vi "Shift left right.vi"(0 "TETRIS BLOCK":u8[][](array[numeric]), 1 "Filled Array":u8[][](array[numeric]), 2 "Move Right":bool) -> (7 "After Shift":u8[][](array[numeric]))   [LabVIEW 2018]
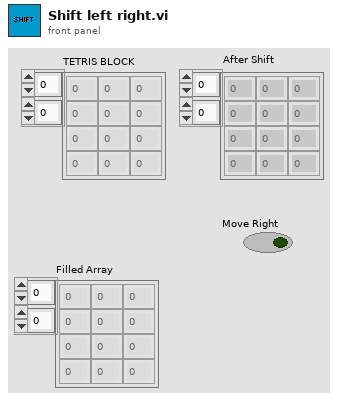
[diagram p1: front panel]
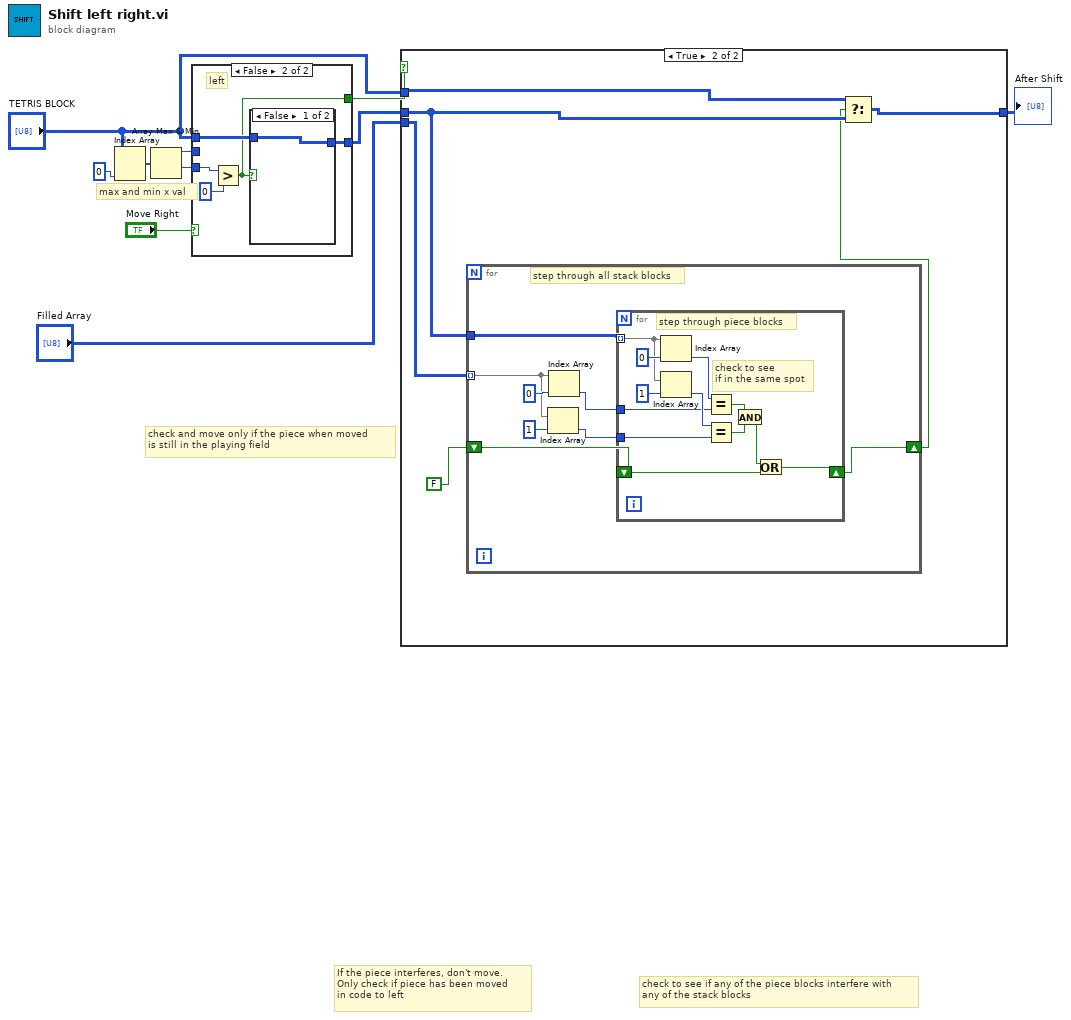
[diagram p0: block diagram]
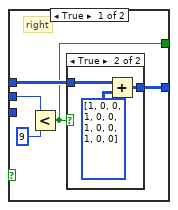
[diagram p3: hidden frame]
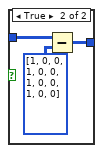
[diagram p5: hidden frame]
diagram:
  # "check to see if any of the piece blocks interfere with \nany of the stack blocks"
  # "max and min x val"
  # "If the piece interferes, don't move.\nOnly check if piece has been moved \nin code to left"
  # "check and move only if the piece when moved\nis still in the playing field"
  n1 = Index Array(array="TETRIS BLOCK", index (col)=0) -> (element=w10:u8[])  [unwired: 1 in]
  n2 = Array Max & Min(array=w10) -> (max value=w8:u8, min value=w1:u8)  [unwired: 2 out]
  n3 = case shown="False" "Move Right" {
    tunnel: w8 -> [w15 _]
    tunnel: "TETRIS BLOCK" -> [w13 w23]
    tunnel: [w12 w22] -> w6
    tunnel: [w11 w21] -> w5
    tunnel: w1 -> [_ w20]
    frame True {
      # "right"
      n4 = Less?(x=w15, y=9) -> (x < y?=w12:bool)
      n5 = case shown="True" w12 {
        tunnel: w13 -> [w16 w18]
        tunnel: [w16 w17] -> w11
        frame False {
        }
        frame True {
          n6 = Add(x=w18, y=i32[][] [[1, 0, 0], [1, 0, 0], [1, 0, 0], [1, 0, 0]]) -> (x+y=w17:i32[][])
        }
      }
    }
    frame False {
      # "left"
      n7 = Greater?(x=w20, y=0) -> (0:w22:bool)
      n8 = case shown="False" w22 {
        tunnel: w23 -> [w25 w27]
        tunnel: [w25 w26] -> w21
        frame False {
        }
        frame True {
          n9 = Subtract(x=w27, y=i32[][] [[1, 0, 0], [1, 0, 0], [1, 0, 0], [1, 0, 0]]) -> (x-y=w26:i32[][])
        }
      }
    }
  }
  n10 = case shown="True" w6 {
    tunnel: w5 -> [w29 w31]
    tunnel: "Filled Array" -> [_ w32]
    tunnel: "TETRIS BLOCK" -> [_ w35]
    tunnel: [w29 w34] -> w2
    frame False {
    }
    frame True {
      n11 = for {
        tunnel: w32 -> [w41] mode=indexing
        shift-right: [w37] -> w30
        shift-left: FALSE -> [w38]
        tunnel: w31 -> [w36]
        # "step through all stack blocks"
        n12 = Index Array(array=w41, index=1) -> (element=w39:u8)
        n13 = Index Array(array=w41, index=0) -> (element=w40:u8)
        n14 = for {
          tunnel: w36 -> [w53] mode=indexing
          tunnel: w40 -> [w50]
          tunnel: w39 -> [w49]
          shift-right: [w45] -> w37
          shift-left: w38 -> [w46]
          # "check to see\nif in the same spot"
          # "step through piece blocks"
          n15 = Index Array(array=w53, index=0) -> (element=w52:i32)
          n16 = Index Array(array=w53, index=1) -> (element=w51:i32)
          n17 = Equal?(x=w52, y=w50) -> (x = y?=w48:bool)
          n18 = Equal?(x=w51, y=w49) -> (x = y?=w47:bool)
          n19 = And(x=w48, y=w47) -> (x .and. y?=w44:bool)
          n20 = Or(x=w44, y=w46) -> (x .or. y?=w45:bool)
        }
      }
      n21 = Select(t=w35, s=w30, f=w31) -> (s? t:f=w34:i32[][])
    }
  }
  "After Shift" <- w2
